vi "Multiple U6 Efunction Loop Example.vi"() -> (0 "error out A":errorcluster)   [LabVIEW 2021]
panel:
  in  "Address B":string="2"
  in  "Address A":string="1"
  out "FIO1 State In B":bool
  in  "DAC0 Voltage B":dbl format="%.3f"
  in  "FIO0 State Out B":bool
  out "Error Message B":string
  out "error out B":errorcluster
  out "AIN0 Voltage B":dbl format="%.6f"
  in  "stop":bool
  in  "Interval (ms)":u32=500
  out "FIO1 State In A":bool
  in  "DAC0 Voltage A":dbl format="%.3f"
  in  "FIO0 State Out A":bool
  out "Error Message A":string
  out "AIN0 Voltage A":dbl format="%.6f"
  # "U3 with LocalID=1:  Sets DAC0, sets FIO0,\nreads AIN0, and reads FIO1."
  # "U3 with LocalID=2:  Sets DAC0, sets FIO0,\nreads AIN0, and reads FIO1."
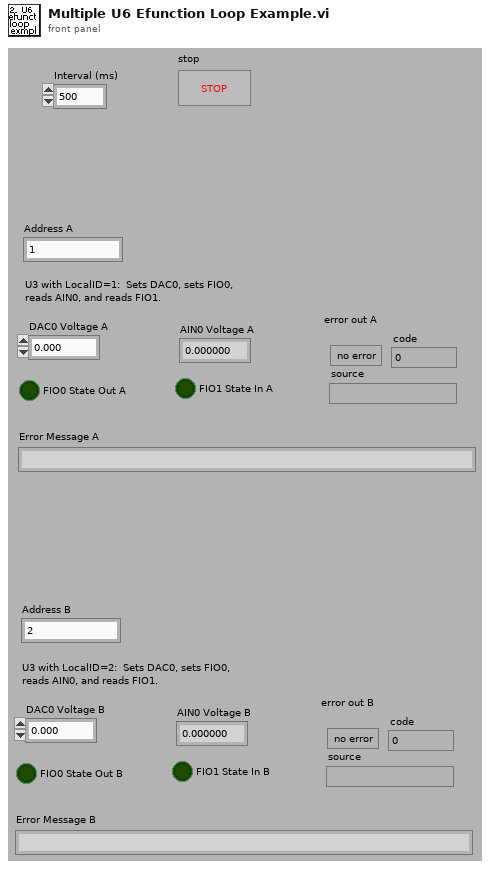
[diagram p1: front panel]
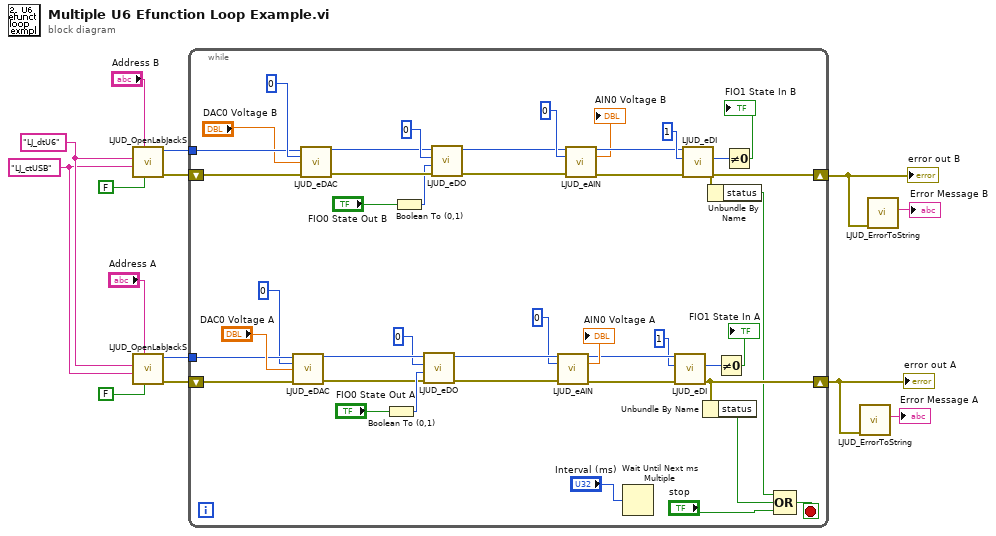
[diagram p0: block diagram]
diagram:
  w1 = "LJ_ctUSB" ("ConnectionType")
  w2 = "LJ_dtU6" ("DeviceType")
  n1 = call "LJUD_OpenLabJackS.vi"("FirstFound"=FALSE, "Address"="Address B", "ConnectionType"=w1, "DeviceType"=w2) -> ("error out"=w5:errorcluster, "Handle"=w6:i32)  [unwired: 5 in, 1 out]
  n2 = call "LJUD_OpenLabJackS.vi"("FirstFound"=FALSE, "Address"="Address A", "ConnectionType"=w1, "DeviceType"=w2) -> ("error out"=w3:errorcluster, "Handle"=w4:i32)  [unwired: 5 in, 1 out]
  n3 = while {
    shift-left: w5 -> [w37]
    shift-right: [w17] -> w9
    tunnel: w6 -> [w27]
    shift-left: w3 -> [w38]
    shift-right: [w39] -> w13
    tunnel: w4 -> [w51]
    stop <- w15 stop-if-true
    n4 = call "LJUD_eDAC.vi"("Handle In"=w51, "Channel"=0, "Voltage"="DAC0 Voltage A", "error in"=w38) -> ("Handle Out"=w49:i32, "error out"=w50:errorcluster)  [unwired: 10 in]
    n5 = call "LJUD_eDAC.vi"("Handle In"=w27, "Channel"=0, "Voltage"="DAC0 Voltage B", "error in"=w37) -> ("Handle Out"=w29:i32, "error out"=w28:errorcluster)  [unwired: 10 in]
    n6 = Boolean To (0,1)(Boolean="FIO0 State Out A") -> (0, 1=w55:i16)
    n7 = Boolean To (0,1)(Boolean="FIO0 State Out B") -> (0, 1=w25:i16)
    n8 = call "LJUD_eDO.vi"("error in"=w50, "State"=w55, "Channel"=0, "Handle In"=w49) -> ("error out"=w48:errorcluster, "Handle Out"=w47:i32)  [unwired: 6 in]
    n9 = call "LJUD_eDO.vi"("error in"=w28, "State"=w25, "Channel"=0, "Handle In"=w29) -> ("error out"=w30:errorcluster, "Handle Out"=w31:i32)  [unwired: 6 in]
    n10 = call "LJUD_eAIN.vi"("Handle In"=w47, "ChannelP"=0, "error in"=w48) -> ("Handle Out"=w43:i32, "Voltage"=→"AIN0 Voltage A":dbl, "error out"=w52:errorcluster)  [unwired: 10 in]
    n11 = call "LJUD_eAIN.vi"("Handle In"=w31, "ChannelP"=0, "error in"=w30) -> ("Handle Out"=w35:i32, "Voltage"=→"AIN0 Voltage B":dbl, "error out"=w26:errorcluster)  [unwired: 10 in]
    n12 = Wait Until Next ms Multiple(millisecond multiple="Interval (ms)") -> ()  [unwired: 1 out]
    n13 = call "LJUD_eDI.vi"("error in"=w52, "Channel"=1, "Handle In"=w43) -> ("error out"=w39:errorcluster, "State"=w56:i32)  [unwired: 6 in, 1 out]
    n14 = call "LJUD_eDI.vi"("error in"=w26, "Channel"=1, "Handle In"=w35) -> ("error out"=w17:errorcluster, "State"=w24:i32)  [unwired: 6 in, 1 out]
    n15 = Unbundle By Name(w39) -> ("status"=w19:bool)
    n16 = Unbundle By Name(w17) -> ("status"=w16:bool)
    n17 = Not Equal To 0?(x=w56) -> (x != 0?=→"FIO1 State In A":bool)
    n18 = Not Equal To 0?(x=w24) -> (x != 0?=→"FIO1 State In B":bool)
    n19 = Compound Arithmetic op=OR(w16, w19, "stop") -> (w15:bool)
  }
  "error out A" <- w13
  "error out B" <- w9
  n20 = call "LJUD_ErrorToString.vi"("error in"=w13) -> ("String"=→"Error Message A":string)  [unwired: 10 in]
  n21 = call "LJUD_ErrorToString.vi"("error in"=w9) -> ("String"=→"Error Message B":string)  [unwired: 10 in]
